vi "Recipe Table to Recipe Steps.vi"(8 "error in (no error)":errorcluster, 11 "Recipe":string[][](table)) -> (0 "error out":errorcluster, 3 "Recipe Steps":refnum<class "Recipe Step.lvclass">[](array[class]))   [LabVIEW 2024, in "Kitchen Actor.lvlib" / "Kitchen Actor.lvclass"]
uses:
  Kitchen Actor.lvclass
  Support/Recipe Step/Recipe Step.lvclass
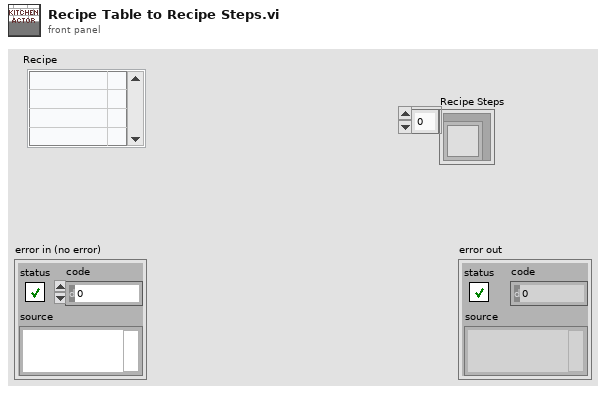
[diagram p1: front panel]
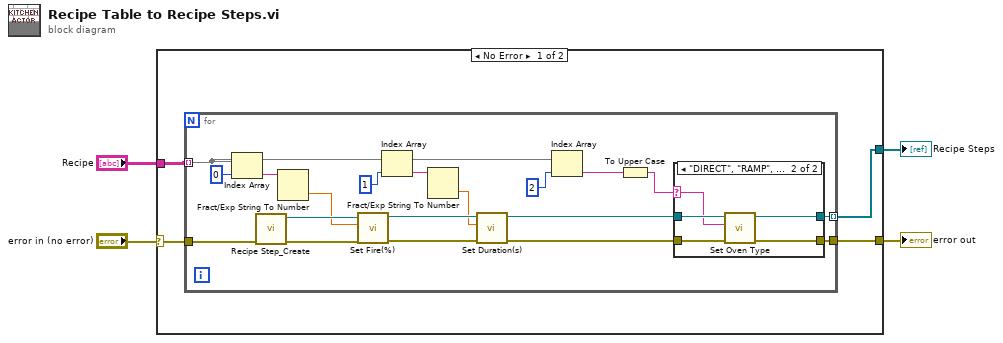
[diagram p0: block diagram]
diagram:
  n1 = case shown="No Error" "error in (no error)" {
    selector: "error in (no error)" -> [w6 w35]
    tunnel: [w5 w35] -> w3
    tunnel: [w8 _] -> w2
    tunnel: "Recipe" -> [w7 _]
    frame No Error {
      n2 = for {
        tunnel: w7 -> [w14] mode=indexing
        tunnel: [w16] -> w8 mode=indexing
        tunnel: [w10] -> w5
        tunnel: w6 -> [w9]
        n3 = Index Array(array=w14, index=0) -> (element=w22:string)
        n4 = call "Recipe Step_Create.vi"("Error In"=w9) -> ("Error Out"=w27:errorcluster, "reference out"=w26:refnum<class "Recipe Step.lvclass">)  [unwired: 9 in]
        n5 = Fract/Exp String To Number(string=w22) -> (number=w18:dbl)  [unwired: 3 in, 1 out]
        n6 = call-dynamic "Set Fire(%).vi"("Error In"=w27, "Fire (%)"=w18, "reference in"=w26) -> ("Error Out"=w25:errorcluster, "reference out"=w24:refnum<class "Recipe Step.lvclass">)  [unwired: 7 in]
        n7 = Index Array(array=w14, index=1) -> (element=w21:string)
        n8 = Fract/Exp String To Number(string=w21) -> (number=w17:dbl)  [unwired: 3 in, 1 out]
        n9 = call-dynamic "Set Duration(s).vi"("Error In"=w25, "Duration (s)"=w17, "reference in"=w24) -> ("Error Out"=w15:errorcluster, "reference out"=w19:refnum<class "Recipe Step.lvclass">)  [unwired: 7 in]
        n10 = Index Array(array=w14, index=2) -> (element=w12:string)
        n11 = To Upper Case(1:w12) -> (0:w11:string)
        n12 = case shown="\"DIRECT\", \"RAMP\", Default" w11 {
          selector: w11 -> [_ w30]
          tunnel: w19 -> [w29 w34]
          tunnel: [w29 w33] -> w16
          tunnel: w15 -> [w28 w32]
          tunnel: [w28 w31] -> w10
          frame "False" {
          }
          frame "DIRECT", "RAMP", Default {
            n13 = call-dynamic "Set Oven Type.vi"("Error In"=w32, "Type"=w30, "reference in"=w34) -> ("Error Out"=w31:errorcluster, "reference out"=w33:refnum<class "Recipe Step.lvclass">)  [unwired: 7 in]
          }
        }
      }
    }
    frame Error {
    }
  }
  "error out" <- w3
  "Recipe Steps" <- w2
